vi "Parse Text-Partial.vi"(8 "Error In":errorcluster) -> (0 "Error Out":errorcluster)   [LabVIEW 2018, in "Tests.lvlib" / "Parser.lvlib"]
uses:
  Parser.lvlib
  src/Toolkit/Public/Tokens/Text/Text.lvclass
  src/Toolkit/Public/Tokens/Partial/Partial.lvclass
  src/Toolkit/Public/Readers/String/String.lvclass
  D:/Users/cfield/Code/Field R&D Services/Mustache/trunk/src/Mustache/Public/Readers/Public/Abstract/Abstract.lvclass
  <vilib>/Utility/LVClass/Get LV Class Name.vi
  src/Toolkit/Public/Tokens/Text/API/Read Content.vi
  <vilib>/addons/_JKI Toolkits/Caraya/classes/Assert/Assert Equal_Variant.vi
  src/Toolkit/Public/Tokens/Keyable/API/Keyable.lvclass
  <vilib>/addons/_JKI Toolkits/Caraya/classes/Test/Test.lvclass
  src/Toolkit/Public/Parser/Parser.lvclass
  <vilib>/addons/_JKI Toolkits/Caraya/classes/Assert/Assert.lvclass
  src/Toolkit/Public/Tokens/Abstract/Abstract.lvclass
  Tests.lvlib
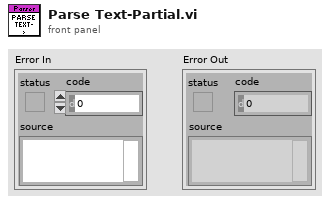
[diagram p1: front panel]
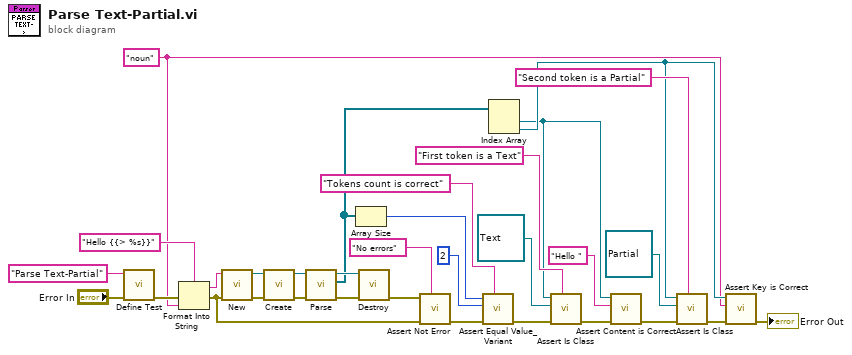
[diagram p0: block diagram]
diagram:
  w4 = "noun" ("String")
  n1 = call <vilib>:"Define Test.vi"("error in (no error)"="Error In", "Label (VI Title)"="Parse Text-Partial") -> ("error out"=w23:errorcluster)  [unwired: 9 in]
  n2 = Format Into String(format string="Hello {{> %s}}", error in=w23, w4) -> (resulting string=w13:string, error out=w15:errorcluster)  [unwired: 1 in]
  n3 = call "New.vi"("Error In"=w15, "String"=w13) -> ("Error Out"=w29:errorcluster, "String"=w30:refnum<class "String.lvclass">)  [unwired: 8 in]
  n4 = call "Create.vi"("Error In"=w29, "Reader"=w30) -> ("Error Out"=w28:errorcluster, "Parser"=w27:refnum<class "Parser.lvclass">)  [unwired: 8 in]
  n5 = call "Parse.vi"("Error In"=w28, "Parser In"=w27) -> ("Error Out"=w25:errorcluster, "Tokens"=w16:refnum<class "Abstract.lvclass">[], "Parser Out"=w26:refnum<class "Parser.lvclass">)  [unwired: 7 in]
  n6 = Array Size(array=w16) -> (size(s)=w19:i32)
  n7 = call "Destroy.vi"("Error In"=w25, "Parser"=w26) -> ("Error Out"=w24:errorcluster)  [unwired: 9 in]
  n8 = call <vilib>:"Assert Not Error.vi"("Label"="No errors", "error in (no error)"=w15, "Not Error?"=w24) -> ("error out"=w21:errorcluster)  [unwired: 8 in]
  n9 = call <vilib>:"Assert Equal Value_Variant.vi"("Label"="Tokens count is correct", "error in (no error)"=w21, "Y"=2 ("size(s)"), "X"=w19) -> ("error out"=w17:errorcluster)  [unwired: 7 in]
  n10 = Index Array(array=w16) -> (element #1=w2:refnum<class "Abstract.lvclass">, element #2=w6:refnum<class "Abstract.lvclass">)  [unwired: 2 in]
  n11 = call "Assert Is Class.vi"("Label"="First token is a Text", "Error In"=w17, "Expected"=refnum<class "Text.lvclass"> refnum ("Mustache.lvlib:Tokens.lvlib:Text.lvclass"), "Actual"=w2) -> ("Error Out"=w12:errorcluster)  [unwired: 7 in]
  n12 = call "Assert Content is Correct.vi"("Error In"=w12, "Expected"="Hello ", "Token"=w2) -> ("Error Out"=w11:errorcluster)  [unwired: 8 in]
  n13 = call "Assert Is Class.vi"("Label"="Second token is a Partial", "Error In"=w11, "Expected"=refnum<class "Partial.lvclass"> refnum ("Mustache.lvlib:Tokens.lvlib:Partial.lvclass"), "Actual"=w6) -> ("Error Out"=w5:errorcluster)  [unwired: 7 in]
  n14 = call "Assert Key is Correct.vi"("Error In"=w5, "Expected"=w4, "Token"=w6) -> ("Error Out"=→"Error Out":errorcluster)  [unwired: 8 in]
